vi "NewLinkSwitch.vi"(6 "Min distance":dbl=2.0, 7 "prev index":i32, 8 "new index":i32, 9 "new element":cluster{"X":dbl, "Y":dbl, "Z":dbl}, 11 "array":T1) -> (3 "array out":T1)   [LabVIEW 2014]
uses:
  Libraries/Map Data Folder/All-Lines.ctl
  Libraries/Map Data Folder/LineCluster.ctl
  Libraries/Map Data Folder/LineConnection.ctl
  Libraries/Map Data Folder/Map Data.lvlib
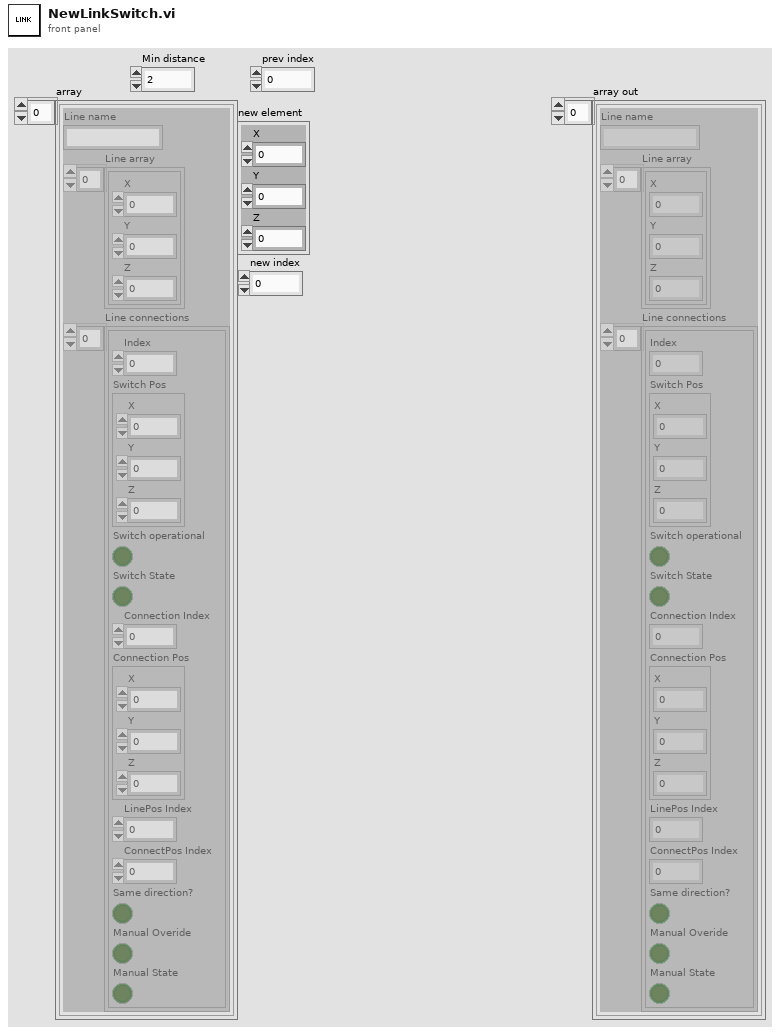
[diagram p1: front panel]
types:
  T1 = typedef "Map Data.lvlib/All-Lines.ctl" = T2[]
  T2 = typedef "Map Data.lvlib/LineCluster.ctl" = cluster{"Line name":string, "Line array":cluster{"X":dbl, "Y":dbl, "Z":dbl}[], "Line connections":T3[]}
  T3 = typedef "Map Data.lvlib/LineConnection.ctl" = cluster{"Index":i32, "Switch Pos":cluster{"X":dbl, "Y":dbl, "Z":dbl}, "Switch operational":bool, "Switch State":bool, "Connection Index":i32, "Connection Pos":cluster{"X":dbl, "Y":dbl, "Z":dbl}, "LinePos Index":i32, "ConnectPos Index":i32, "Same direction?":bool, "Manual Overide":bool, "Manual State":bool}
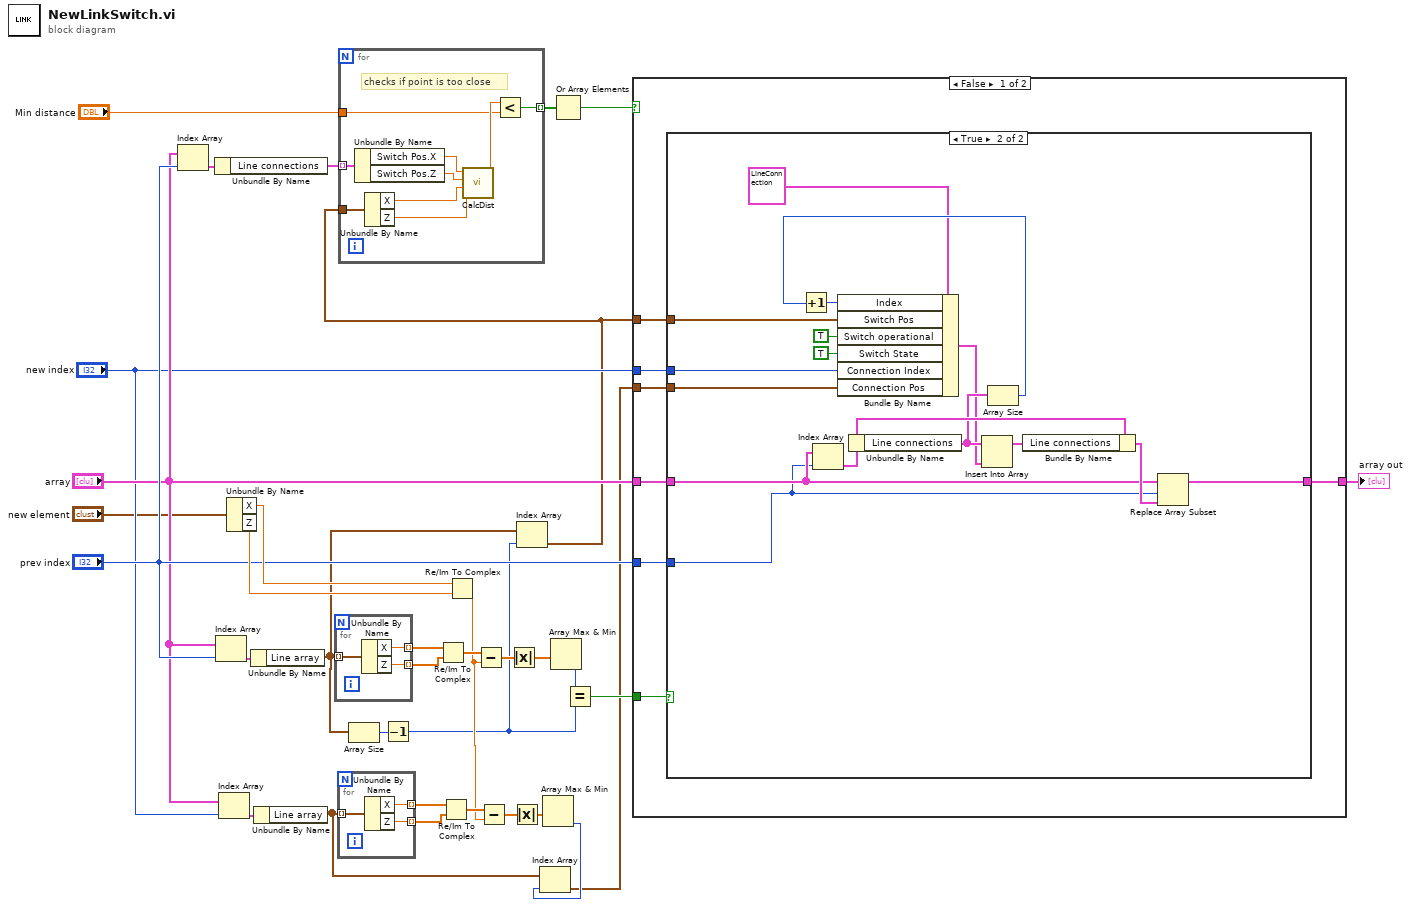
[diagram p0: block diagram]
diagram:
  n1 = Index Array(array="array", index="prev index") -> (element=w21:T2)
  n2 = Unbundle By Name(w21) -> ("Line connections"=w20:T3[])
  n3 = Index Array(array="array", index="prev index") -> (element=w26:T2)
  n4 = Index Array(array="array", index="new index") -> (element=w8:T2)
  n5 = Unbundle By Name("new element") -> ("X"=w25:dbl, "Z"=w24:dbl)
  n6 = Unbundle By Name(w26) -> ("Line array"=w3:cluster{"X":dbl, "Y":dbl, "Z":dbl}[])
  n7 = Unbundle By Name(w8) -> ("Line array"=w7:cluster{"X":dbl, "Y":dbl, "Z":dbl}[])
  n8 = for {
    tunnel: [w37] -> w30 mode=indexing
    tunnel: [w36] -> w29 mode=indexing
    tunnel: w3 -> [w35] mode=indexing
    n9 = Unbundle By Name(w35) -> ("X"=w37:dbl, "Z"=w36:dbl)
  }
  n10 = for {
    tunnel: [w40] -> w14 mode=indexing
    tunnel: [w39] -> w15 mode=indexing
    tunnel: w7 -> [w38] mode=indexing
    n11 = Unbundle By Name(w38) -> ("X"=w40:dbl, "Z"=w39:dbl)
  }
  n12 = Array Size(array=w3) -> (size(s)=w33:i32)
  n13 = Decrement(x=w33) -> (x-1=w4:i32)
  n14 = Re/Im To Complex(1:w29, 2:w30) -> (0:w28:cdb[])
  n15 = Re/Im To Complex(1:w15, 2:w14) -> (0:w16:cdb[])
  n16 = Re/Im To Complex(1:w24, 2:w25) -> (0:w11:cdb)
  n17 = Subtract(x=w28, y=w11) -> (x-y=w32:cdb[])
  n18 = Subtract(x=w16, y=w11) -> (x-y=w12:cdb[])
  n19 = Absolute Value(x=w32) -> (abs(x)=w31:dbl[])
  n20 = Absolute Value(x=w12) -> (abs(x)=w13:dbl[])
  n21 = Index Array(array=w3, index=w4) -> (element=w1:cluster{"X":dbl, "Y":dbl, "Z":dbl})
  n22 = for {
    tunnel: w20 -> [w49] mode=indexing
    tunnel: w1 -> [w48]
    tunnel: "Min distance" -> [w46]
    tunnel: [w41] -> w18 mode=indexing
    # "checks if point is too close"
    n23 = Unbundle By Name(w49) -> ("Switch Pos.X"=w45:dbl, "Switch Pos.Z"=w44:dbl)
    n24 = Unbundle By Name(w48) -> ("X"=w43:dbl, "Z"=w42:dbl)
    n25 = call "CalcDist.vi"("Y2"=w42, "X2"=w43, "Y1"=w44, "X1"=w45) -> ("Distance"=w47:dbl)  [unwired: 7 in]
    n26 = Less?(x=w47, y=w46) -> (x < y?=w41:bool)
  }
  n27 = Array Max & Min(array=w13) -> (min index (indices)=w6:i32)  [unwired: 3 out]
  n28 = Index Array(array=w7, index=w6) -> (element=w5:cluster{"X":dbl, "Y":dbl, "Z":dbl})
  n29 = Array Max & Min(array=w31) -> (min index (indices)=w27:i32)  [unwired: 3 out]
  n30 = Or Array Elements(Boolean array=w18) -> (logical OR=w17:bool)
  n31 = Equal?(x=w27, y=w4) -> (x = y?=w23:bool)
  n32 = case shown="False" w17 {
    tunnel: w1 -> [w56 _]
    tunnel: "new index" -> [w55 _]
    tunnel: [w54 w74] -> w34
    tunnel: w23 -> [w53 _]
    tunnel: "array" -> [w52 w74]
    tunnel: "prev index" -> [w51 _]
    tunnel: w5 -> [w50 _]
    frame False {
      n33 = case shown="True" w53 {
        tunnel: w56 -> [_ w67]
        tunnel: w55 -> [_ w66]
        tunnel: [w57 w63] -> w54
        tunnel: w52 -> [w57 w62]
        tunnel: w51 -> [_ w61]
        tunnel: w50 -> [_ w60]
        frame False {
        }
        frame True {
          n34 = Index Array(array=w62, index=w61) -> (element=w73:T2)
          n35 = Unbundle By Name(w73) -> ("Line connections"=w70:T3[])
          n36 = Array Size(array=w70) -> (size(s)=w69:i32)
          n37 = Increment(x=w69) -> (x+1=w68:i32)
          n38 = Bundle By Name(cluster=T3 {"Index"=0, "Switch Pos"={"X"=0.0, "Y"=0.0, "Z"=0.0}, "Switch operational"=FALSE, "Switch State"=FALSE, "Connection Index"=0, "Connection Pos"={"X"=0.0, "Y"=0.0, "Z"=0.0}, "LinePos Index"=0, "ConnectPos Index"=0, "Same direction?"=FALSE, "Manual Overide"=FALSE, "Manual State"=FALSE}, "Index"=w68, "Switch Pos"=w67, "Switch operational"=TRUE, "Switch State"=TRUE, "Connection Index"=w66, "Connection Pos"=w60) -> (w59:T3)
          n39 = Insert Into Array(array=w70, new element=w59) -> (w72:T3[])  [unwired: 1 in]
          n40 = Bundle By Name(cluster=w73, "Line connections"=w72) -> (w71:T2)
          n41 = Replace Array Subset(array=w62, new element=w71, index=w61) -> (w63:T1)
        }
      }
    }
    frame True {
    }
  }
  "array out" <- w34
